vi "main.vi"() -> ()   [LabVIEW 2012]
panel:
  in  "stop":bool
  out "Waveform Chart":dbl(graph)
  # "This is the main VI of our program.  This VI does not do anything special,\nbut it does let you know when the splash screen VI finishes running."
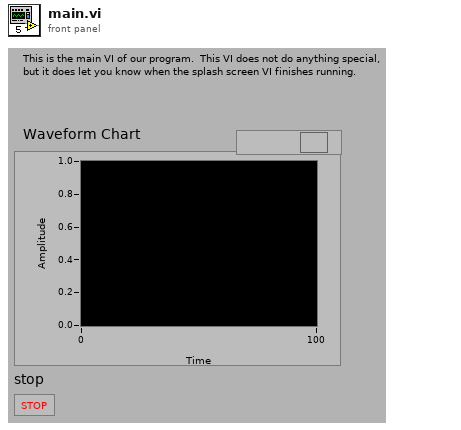
[diagram p1: front panel]
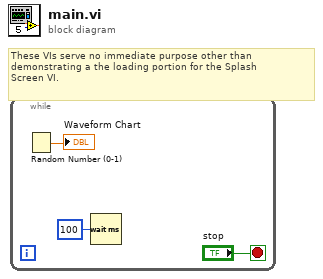
[diagram p0: block diagram]
diagram:
  # "These VIs serve no immediate purpose other than \ndemonstrating a the loading portion for the Splash \nScreen VI."
  n1 = while {
    stop <- "stop" stop-if-true
    n2 = Random Number (0-1)() -> (number: 0 to 1=→"Waveform Chart":dbl)
    n3 = Wait (ms)(milliseconds to wait=u32 100) -> ()  [unwired: 1 out]
  }
